vi "ReadWrite.Data.Read.vi"(8 "error in (no error)":errorcluster, 10 "timeout ms":i32, 11 "Ref":T1) -> (0 "error out":errorcluster, 1 "Timeout?":bool, 2 "Data":dbl[](array[numeric]), 3 "Detect?":bool[](array[boolean]))   [LabVIEW 2015, in "Data Access Engine.lvlib" / "Data Access Engine.lvclass"]
uses:
  Data Access Engine.lvclass
  Types/ReadWrite.DVR.ctl
  Access Type Classes/ReadWrite/ReadWrite.lvclass
  Access Type Classes/ReadWrite/ReadWrite.lvclass/ReadWrite.ctl
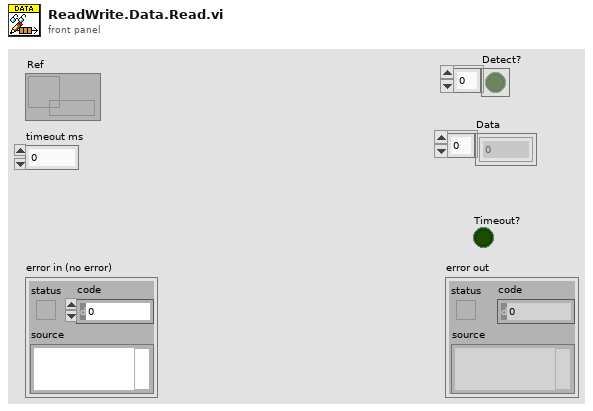
[diagram p1: front panel]
types:
  T1 = typedef "Data Access Engine.lvlib/Data Access Engine.lvclass/ReadWrite.DVR.ctl" = refnum<data-value>
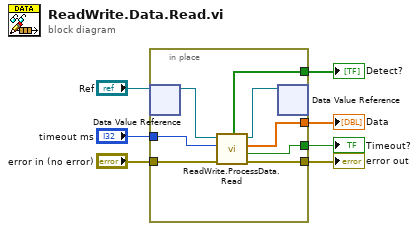
[diagram p0: block diagram]
diagram:
  n1 = in-place {
    in-place-border: "error in (no error)" -> [w15]
    in-place-border: [w14] -> w6
    in-place-border: "timeout ms" -> [w12]
    in-place-border: [w10] -> w3
    in-place-border: [w9] -> w2
    in-place-border: [w8] -> w1
    n2 = in-place-dvr #1("Ref") -> (w13:refnum<class "ReadWrite.lvclass">)  [unwired: 1 out]
    n3 = call "ReadWrite.ProcessData.Read.vi"("error in (no error)"=w15, "timeout ms"=w12, "ReadWrite in"=w13) -> ("error out"=w14:errorcluster, "Timeout?"=w9:bool, "Values"=w10:dbl[], "ReadWrite out"=w11:refnum<class "ReadWrite.lvclass">, "Detect?"=w8:bool[])  [unwired: 4 in]
    n4 = in-place-dvr #1(w11) -> ()  [unwired: 2 out]
  }
  "error out" <- w6
  "Data" <- w3
  "Timeout?" <- w2
  "Detect?" <- w1
